vi "dfd_QMF Lattice Analysis Bank with State (Array).vi"(6 "state in":cluster{"state":dbl[]}[](array[cluster]), 8 "error in (no error)":errorcluster, 10 "filter bank in":T1={"mBank_Filters"=[], " mBank_#Bands"=2, "mBank_ProcMethod"=enum."General", "mBank_Coeffs"=[], "mBank_Gain"=1.0, "mBank_Type"=0} {"mBank_Type" items=["Uniform", "Non-Uniform"]; "mBank_Filters"."mMRate_SumWl" min=1 max=32 step=1; "mBank_Filters"."mMRate_InputIwl" min=1 max=32 step=1; "mBank_Filters"."mMRate_GainWl" min=1 max=32 step=1; "mBank_Filters"."mMRate_OutputWl" min=1 max=32 step=1; "mBank_Filters"."mMRate_InputWl" min=1 max=32 step=1; "mBank_Filters"."mMRate_CoefWl" min=1 max=32 step=1; "mBank_Filters"."mMRate_Mode" items=["Default"=-1, "No Rate Change"=0, "Interpolation"=1, "Decimation"=2, "Interpolated"=3, "Rational"=4]}, 11 "x":dbl[](array[numeric]) format="%.2f") -> (0 "error out":errorcluster, 2 "highpass channel":dbl[](array[numeric]) format="%.2f", 3 "lowpass channel":dbl[](array[numeric]) format="%.2f", 4 "state out":cluster{dbl[]}[](array[cluster]))   [LabVIEW 2017, in "NI_DigFilter_FilterBank.lvlib"]
uses:
  <vilib>/addons/Digital Filter Design/NI_DigFilter_FilterBank.lvlib
  <vilib>/addons/Digital Filter Design/FilterBank.llb/Object/DFD Bank Obj.ctl
  <vilib>/addons/Digital Filter Design/_Objects.llb/DFD Multirate Filter Obj.ctl
  <vilib>/addons/Digital Filter Design/_Objects.llb/DFD Multirate Mode.ctl
  <vilib>/addons/Digital Filter Design/_Objects.llb/DFD Coef Norm Type.ctl
  <vilib>/addons/Digital Filter Design/_Objects.llb/DFD Round-off Mode.ctl
  <vilib>/addons/Digital Filter Design/_Objects.llb/DFD FXP MRate Multiply Mode.ctl
  <vilib>/addons/Digital Filter Design/FilterBank.llb/Object/DFD Filter Bank Processing Method.ctl
  <vilib>/addons/Digital Filter Design/FilterBank.llb/Object/DFD Filter Bank Type.ctl
  <vilib>/addons/Digital Filter Design/_Misc.llb/dfd_Error Cluster From Error Code (Scalar).vi
  <vilib>/addons/Digital Filter Design/NI_DigFilterLicensed.lvlib
  <resource>/LVDFD.dll
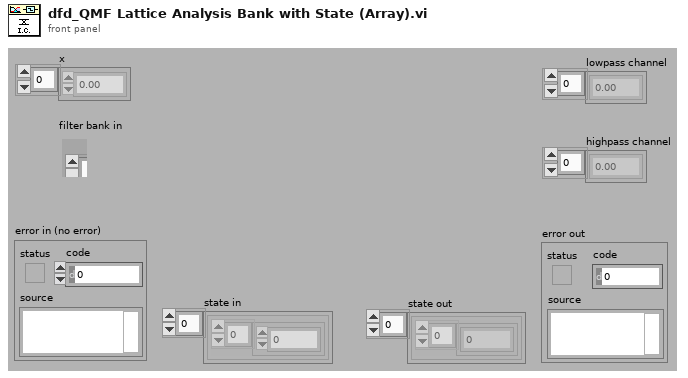
[diagram p1: front panel]
types:
  T1 = typedef "NI_DigFilter_FilterBank.lvlib/DFD Bank Obj.ctl" = cluster{"mBank_Filters":T2[], " mBank_#Bands":i32, "mBank_ProcMethod":T7, "mBank_Coeffs":dbl[], "mBank_Gain":dbl, "mBank_Type":T8}
  T2 = typedef "NI_DigFilterLicensed.lvlib/DFD Multirate Filter Obj.ctl" = cluster{"mMRate_Structure":enum16{"CIC", "FIR", "IIR", "Lattice"}, "mMRate_Mode":T3, "mMRate_Factor":i32, "mMRate_FIRParams":cluster{"mMRate_FIR_H":dbl[], "mMRate_FIR_IsNyquist?":bool, "mMRate_FIR_IsSymmetric?":bool}, "mMRate_CICParams":cluster{"mMRate_CIC_#Stage":i32, "mMRate_CIC_Lag":i32, "mMRate_CIC_Type":enum16{"Lowpass", "Highpass"}}, "mMRate_Order":i32, "mMRate_Version":string, "mMRate_Comments":string, "mMRate_RationalFactor":cluster{"mMRate_L":i32, "mMRate_M":i32}, "mMRate_Fs":dbl, "mMRate_Quantized?":bool, "mMRate_QFilterGain":dbl, "mMRate_CoefWl":i16, "mMRate_Scaling":cluster{"mMRate_ScaleByPowerOf2?":bool, "mMRate_ScaleType":T4}, "mMRate_InputWl":i16, "mMRate_OutputWl":i16, "mMRate_OutputMode":T5, "mMRate_MultMode":T6, "mMRate_BitPruning":bool, "mMRate_GainWl":i16, "mMRate_OutputFwl":i16, "mMRate_SumIwl":i16, "mMRate_InputIwl ":i16, "mMRate_SumWl":i16, "mMRate_CoefIwl":i16}
  T3 = typedef "NI_DigFilterLicensed.lvlib/DFD Multirate Mode.ctl" = i16
  T4 = typedef "NI_DigFilterLicensed.lvlib/DFD Coef Norm Type.ctl" = enum16{"No Norm", "Time Domain 1-Norm", "Time Domain 2-Norm", "Time Domain Inf-Norm"}
  T5 = typedef "NI_DigFilterLicensed.lvlib/DFD Round-off Mode.ctl" = enum16{"Nearest", "Truncation"}
  T6 = typedef "NI_DigFilterLicensed.lvlib/DFD FXP MRate Multiply Mode.ctl" = enum16{"Truncated", "Full"}
  T7 = typedef "NI_DigFilter_FilterBank.lvlib/DFD Filter Bank Processing Method.ctl" = enum16{"General", "2-Band QMF Lattice", "Cosine-Modulated"}
  T8 = typedef "NI_DigFilter_FilterBank.lvlib/DFD Filter Bank Type.ctl" = u16
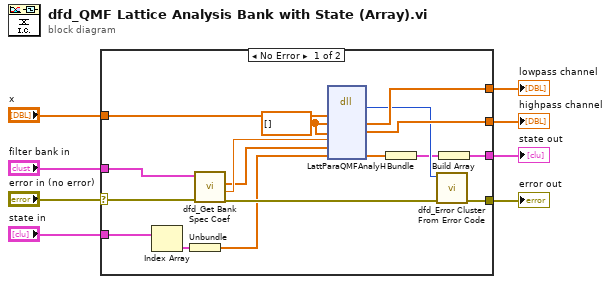
[diagram p0: block diagram]
diagram:
  n1 = case shown="No Error" "error in (no error)" {
    selector: "error in (no error)" -> [w9 w26]
    tunnel: "x" -> [w23 _]
    tunnel: [w25 w26] -> w7
    tunnel: [w24 _] -> w6
    tunnel: [w22 _] -> w5
    tunnel: "state in" -> [w18 _]
    tunnel: [w15 _] -> w3
    tunnel: "filter bank in" -> [w10 _]
    frame No Error {
      w20 = dbl[] [] ("outputDatay1H")
      n2 = Index Array(array=w18) -> (element=w19:cluster{"state":dbl[]})  [unwired: 1 in]
      n3 = Unbundle(w19) -> ("state"=w11:dbl[])
      n4 = call <vilib>:"dfd_Get Bank Spec Coef.vi"("error in (no error)"=w9, "bank in"=w10) -> ("error out"=w12:errorcluster, "gain"=w14:dbl, "coefficients"=w13:dbl[])  [unwired: 4 in, 3 out]
      n5 = dll-call lib="C:/Program Files/National Instruments/LabVIEW 2017/resource/LVDFD.*" fn="LattParaQMFAnalyH"("inputDataH"=w23, "outputDatay1H"=w20, "outputDatay2H"=w20, "gainH"=w14, "coeffKH"=w13, "initialStatesH"=w11) -> ("return type"=w21:i32, "outputDatay1H"=w24:dbl[], "outputDatay2H"=w22:dbl[], "initialStatesH"=w17:dbl[])  [unwired: 6 in, 2 out]
      n6 = Bundle("initialStatesH"=w17) -> (w16:cluster{"initialStatesH":dbl[]})  [unwired: 1 in]
      n7 = call-poly <vilib>:"dfd_Error Cluster From Error Code.vi"("error in (no error)"=w12, "error code (0)"=w21) -> ("error out"=w25:errorcluster)  [unwired: 9 in]
      n8 = Build Array(w16) -> (w15:cluster{"initialStatesH":dbl[]}[])
    }
    frame Error {
    }
  }
  "lowpass channel" <- w6
  "error out" <- w7
  "highpass channel" <- w5
  "state out" <- w3
